vi "Admittance_control_30_07_2017adding_admittance_to_impedance_control.vi"() -> ()   [LabVIEW 2016]
uses:
  <vilib>/Platform/TimedLoop/XDataNode/timing_clust.ctl
  <vilib>/Platform/TimedLoop/XDataNode/nitl_modes.ctl
  <vilib>/Platform/TimedLoop/XDataNode/wakeup.ctl
  <vilib>/Platform/TimedLoop/XDataNode/loadnilvce.vi
  <vilib>/Motion/Express/_s/nimc.ax.power.power.axis.vi
  <vilib>/Motion/Express/_s/nimc.fb.read.readExecutionData.axis.vi
  <vilib>/Motion/Express/_s/nimc.fb.stopMove.stop.axis.modeDecelerate.vi
  <vilib>/Motion/Express/_s/nimc.fb.straightLineMove.startStraightLineMove.axis.modeVelocity.0.vi
  <vilib>/Motion/Express/_s/nimc.fb.resetPosition.resetPosition.axis.vi
  <vilib>/Motion/Express/_s/nimc.ex.power.power.axis.vi
  <vilib>/platform/TimedLoop/XDataNode/XDataNode.xnode
  <vilib>/Motion/BlockNode/FB.NIMotion.xnode
  <vilib>/Platform/TimedLoop/XDataNode/XDNodeRunTimeDep.lvlib
panel:
  in  "Exogenouse Force Req CCW":dbl=0.3 format="%#_13g"
  in  "Exogenouse Force Req CW":dbl=-0.3 format="%#_13g"
  in  "Velocity Gain":dbl=0.25 format="%#_12g"
  in  "Arm Stop Torque CCW":dbl=0.25 format="%#_12g"
  in  "Arm Stop Torque CW":dbl=0.25 format="%#_12g"
  out "Exogenous torque, Nm":dbl format="%.3f"
  out "Exogenouse Torque":dbl(knob) scale=-1.0..2.0
  out "Adjusted Velocity, Rad/s":dbl format="%.3f"
  out "Adjusted Velocity":dbl(knob) scale=-1.0..2.0
  in  "Reset Position":bool
  in  "Velocity Setpoint, Rad/s":dbl=0.25 format="%#_12g"
  out "Raw Torque Value":dbl(knob) scale=-3.0..3.0
  out "Position":dbl(knob) scale=-1.0..1.0
  out "Velocity":dbl(knob) scale=-1.0..5.0
  out "Load Cell":dbl(knob) scale=0.0..10.0
  in  "Move to Position?":bool
  out "Load cell, V":dbl format="%.3f"
  out "Raw motor torque, Nm":dbl format="%.3f"
  out "Velocity, Rad/s":dbl format="%.3f"
  out "Position, [0-1]":dbl format="%.3f"
  in  "STOP VI":bool
  in  "Enable Axis \nControl":bool
  in  "Enable Motor \nDrive":bool
  in  "EMERGENCY MOTOR STOP":bool
  # "Raw Data from System"
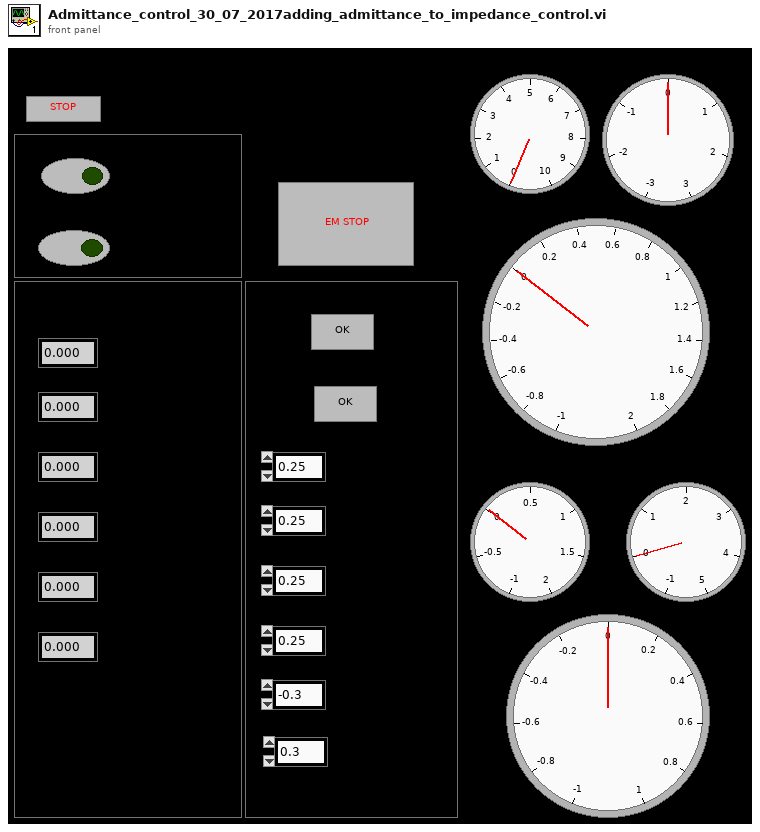
[diagram p1: front panel]
types:
  T1 = typedef "XDNodeRunTimeDep.lvlib/timing_clust.ctl" = cluster{"Expected End [f-1]":u64, "Actual End [f-1]":u64, "Finished Late? [f-1]":bool, "Expected End [i-1]":u64, "Actual End [i-1]":u64, "Finished Late? [i-1]":bool, "Expected Start [i]":u64, "Actual Start [i]":u64, "Expected Start [f]":u64, "Actual Start [f]":u64, "Source Name":string, "Structure Name":string, "Period":i64, "Deadline":i64, "Offset":i64, "Start":i64, "Priority":i32, "Timeout":i32, "Mode":T2, "Wakeup Reason":T3, "Error":errorcluster, "Source Type":string, "Secondary Source Type":string, "Global End Time":u64, "Global Start Time":u64, "Frame Duration":u64, "Iteration Duration":u64, "Assigned CPU":i32, "I/O Scan Engine Mode":u32}
  T2 = typedef "XDNodeRunTimeDep.lvlib/nitl_modes.ctl" = enum32{"No Change", "Process missed periods, maintain original phase", "Discard missed periods, maintain original phase", "Process missed periods, ignore original phase", "Discard missed periods, ignore original phase"}
  T3 = typedef "XDNodeRunTimeDep.lvlib/wakeup.ctl" = enum32{"Normal", "Aborted", "Asynchronous wakeup", "Timing source error", "Timed loop error", "Timeout"}
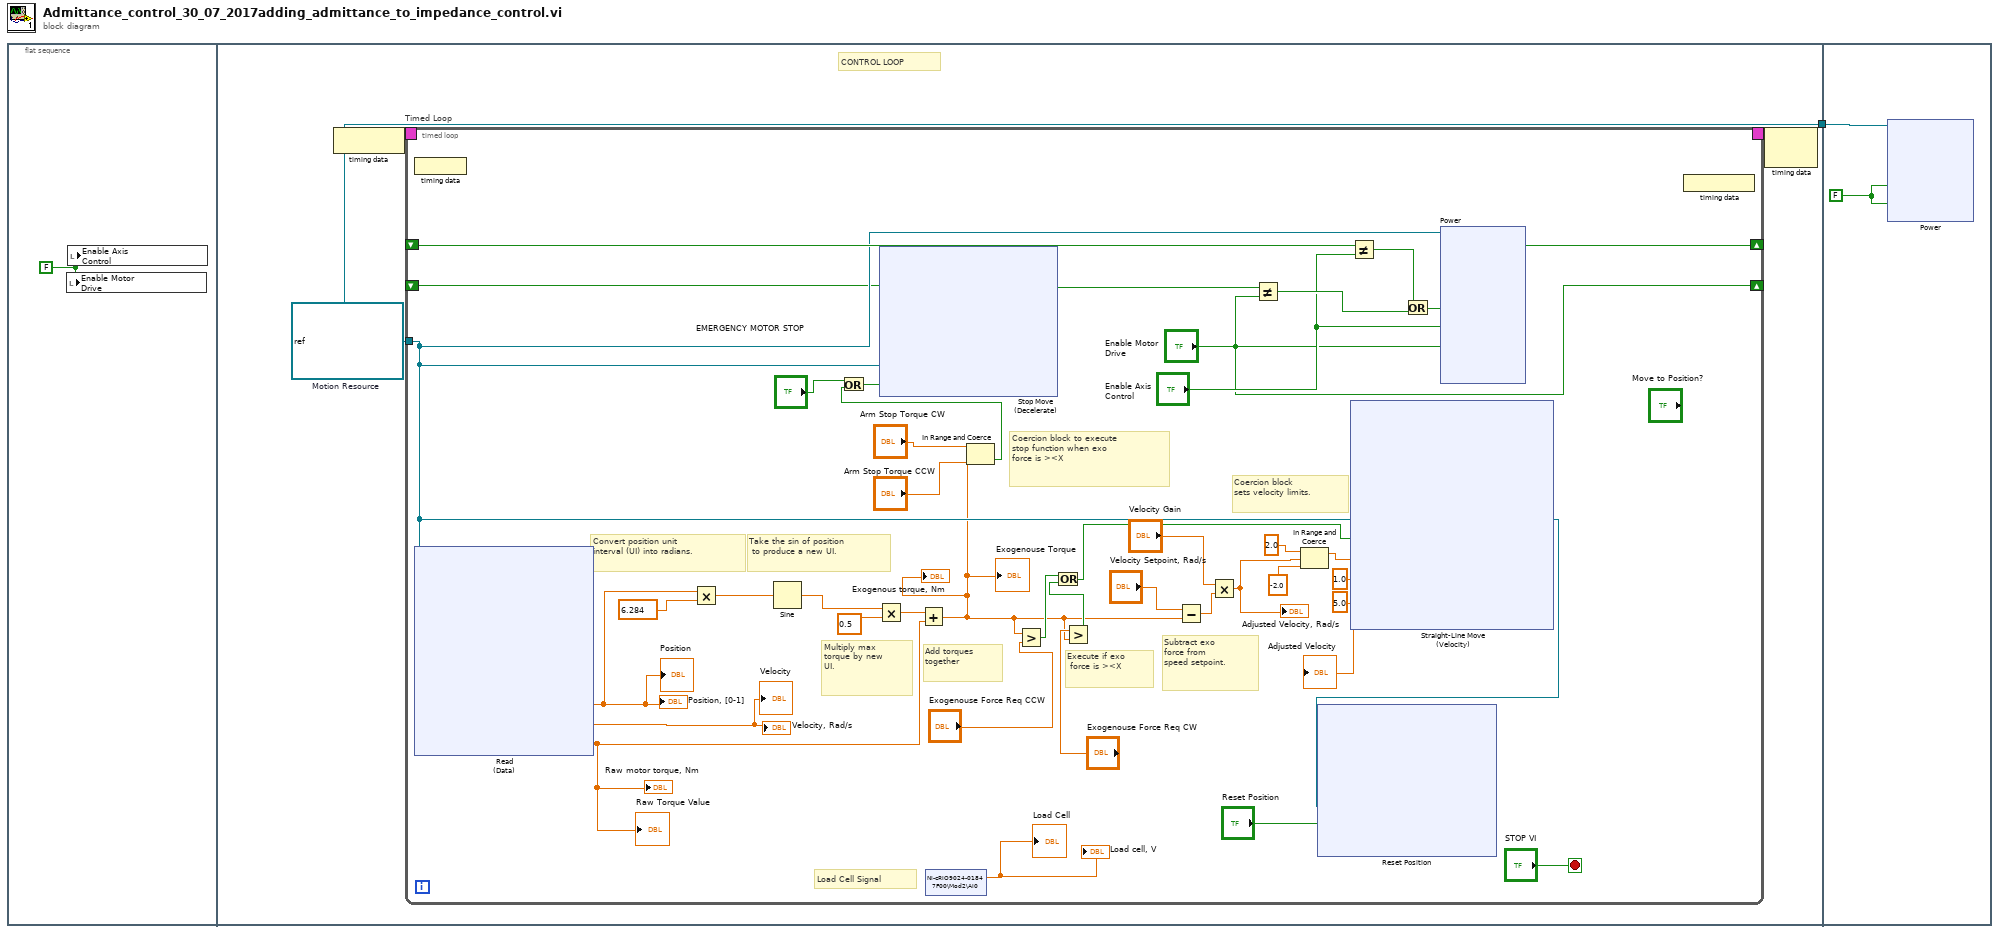
[diagram p0: block diagram]
diagram:
  n1 = flat-sequence {
    tunnel: [w5] -> w1
    tunnel: w1 -> [w123]
    frame #0 {
      w2 = FALSE
      n2 = local write "Enable Motor \nDrive"(w2) -> ()
      n3 = local write "Enable Axis \nControl"(w2) -> ()
    }
    frame #1 {
      w5 = refnum<k21> "nism://NI-cRIO9024-01847F00/Axis 1"  # Motion Resource
      # "CONTROL LOOP"
      n4 = node-c288() -> (w4:T1)
      n5 = timed-loop "Timed Loop" {
        tunnel: w5 -> [w37]
        timing: w4 -> [_]
        timing-out: [_] -> w3
        shift-right: ["Enable Axis \nControl"] -> _
        shift-left: _ -> [w44]
        shift-right: ["Enable Motor \nDrive"] -> _
        shift-left: _ -> [w31]
        stop <- "STOP VI" stop-if-true
        # "Coercion block to execute\nstop function when exo \nforce is ><X"
        # "Coercion block\nsets velocity limits."
        # "Subtract exo\nforce from\nspeed setpoint."
        # "Execute if exo\n force is ><X"
        # "Add torques\ntogether"
        # "Multiply max \ntorque by new\nUI."
        # "Take the sin of position\n to produce a new UI."
        # "Convert position unit \ninterval (UI) into radians."
        # "Load Cell Signal"
        n6 = node-c288() -> ()  [unwired: 1 in]
        n7 = xnode "Read\n(Data)"("resource"=w37) -> ("position"=w7:dbl, "torque"=w23:dbl, "velocity"=→"Velocity, Rad/s" →"Velocity":dbl)  [unwired: 1 in, 3 out]
        "Position, [0-1]" <- w7
        "Raw motor torque, Nm" <- w23
        "Position" <- w7
        "Raw Torque Value" <- w23
        n8 = Multiply(x=w7, y=6.284) -> (x*y=w6:dbl)
        n9 = Sine(x=w6) -> (sin(x)=w24:dbl)
        n10 = Multiply(x=w24, y=0.5) -> (x*y=w22:dbl)
        n11 = Add(x=w22, y=w23) -> (x+y=w8:dbl)
        "Exogenouse Torque" <- w8
        "Exogenous torque, Nm" <- w8
        n12 = shared-variable "NI-cRIO9024-01847F00\\Mod2\\AI0"() -> (→"Load cell, V" →"Load Cell":dbl)  [unwired: 1 in, 1 out]
        n13 = In Range and Coerce(upper limit="Arm Stop Torque CW", x=w8, lower limit="Arm Stop Torque CCW") -> (In Range?=w12:bool)  [unwired: 1 out]
        n14 = Or(x="EMERGENCY MOTOR STOP", y=w12) -> (x .or. y?=w16:bool)
        n15 = xnode "Stop Move\n(Decelerate)"("resource"=w37, "execute"=w16) -> ()  [unwired: 1 in, 3 out]
        n16 = Greater?(x=w8, y="Exogenouse Force Req CCW") -> (0:w18:bool)
        n17 = Greater?(x="Exogenouse Force Req CW", y=w8) -> (0:w19:bool)
        n18 = Or(x=w18, y=w19) -> (x .or. y?=w9:bool)
        n19 = Subtract(x="Velocity Setpoint, Rad/s", y=w8) -> (x-y=w14:dbl)
        n20 = Multiply(x="Velocity Gain", y=w14) -> (x*y=w15:dbl)
        "Adjusted Velocity, Rad/s" <- w15
        n21 = Not Equal?(x=w31, y="Enable Motor \nDrive") -> (x != y?=w42:bool)
        n22 = In Range and Coerce(upper limit=2.0, x=w15, lower limit=-2.0) -> (coerced(x)=w27:dbl)  [unwired: 1 out]
        "Adjusted Velocity" <- w27
        n23 = Not Equal?(x=w44, y="Enable Axis \nControl") -> (x != y?=w43:bool)
        n24 = xnode "Straight-Line Move\n(Velocity)"("resource"=w37, "execute"=w9, "velocity"=w27, "acceleration"=1.0, "deceleration"=5.0) -> ("resource out"=w34:refnum<k21>)  [unwired: 1 in, 2 out]
        n25 = xnode "Reset Position"("resource"=w34, "execute"="Reset Position") -> ()  [unwired: 2 in, 3 out]
        n26 = Or(x=w43, y=w42) -> (x .or. y?=w41:bool)
        n27 = xnode ("Power")("execute"=w41, "enable axis"="Enable Axis \nControl", "enable drive"="Enable Motor \nDrive", "resource"=w37) -> ()  [unwired: 1 in, 6 out]
        n28 = node-c288() -> ()  [unwired: 1 out]
      }
      n29 = node-c288(w3) -> ()  [unwired: 1 out]
    }
    frame #2 {
      w124 = FALSE
      n30 = xnode ("Power")("enable axis"=w124, "enable drive"=w124, "resource"=w123) -> ()  [unwired: 1 in, 2 out]
    }
  }
